vi "v0.01.vi"() -> ()   [LabVIEW 2021]
uses:
  C/Program Files/National Instruments/LabVIEW 2024/instr.lib/lvserial/lvserial.lvlib
panel:
  out "XY Graph":cluster{"X":dbl, "Y":dbl}[](graph)
  out "Imag":i32[](array[numeric])
  out "Real":i32[](array[numeric])
  out "F":dbl[](array[numeric])
  out "x/y":dbl
  in  "Step":i32
  in  "Stop":i32
  in  "Start":i32
  out "Array 3":string[](array[string])
  out "string read":string
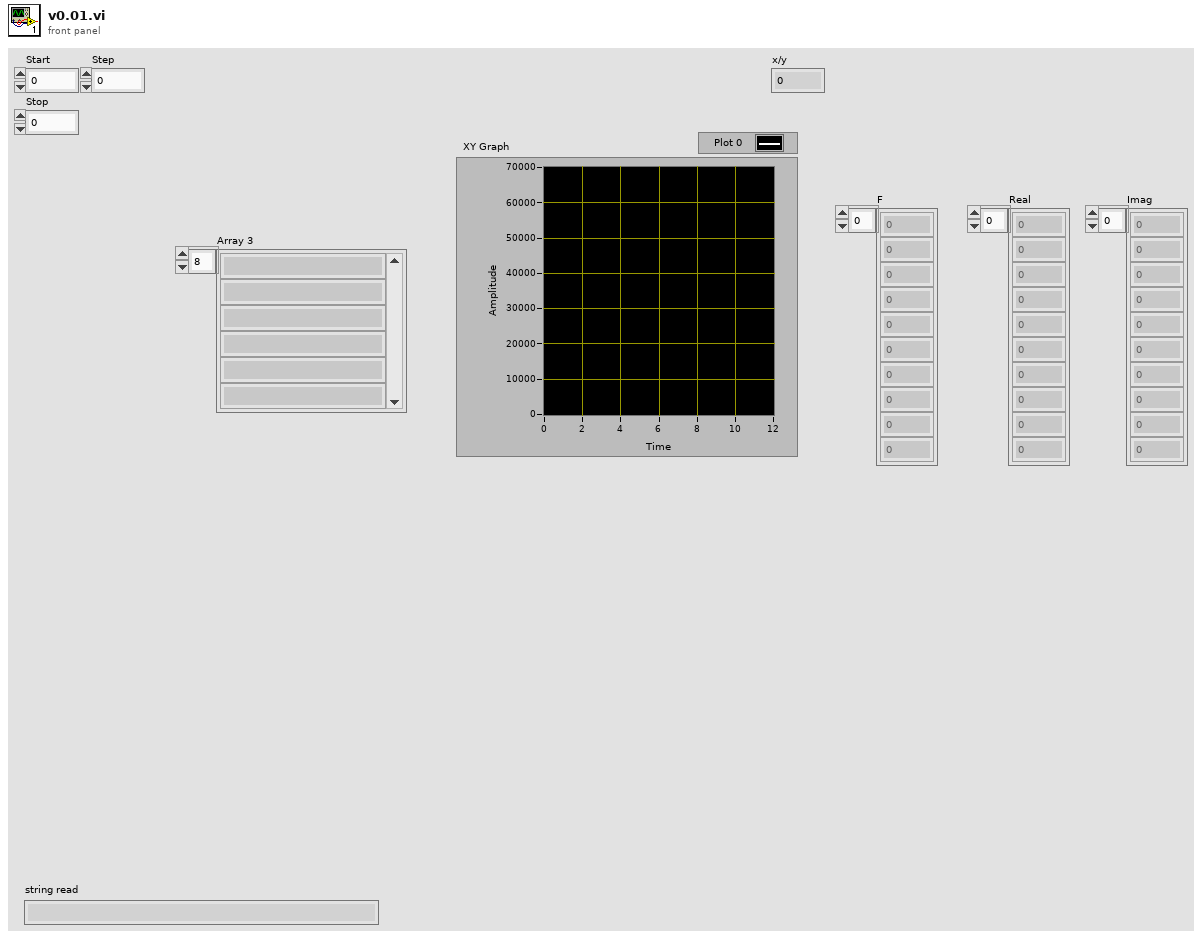
[diagram p1: front panel]
types:
  T1 = cluster{"Baud Rate":u32, "Data Bits":u16, "Parity":u16, "Stop Bits":u16}
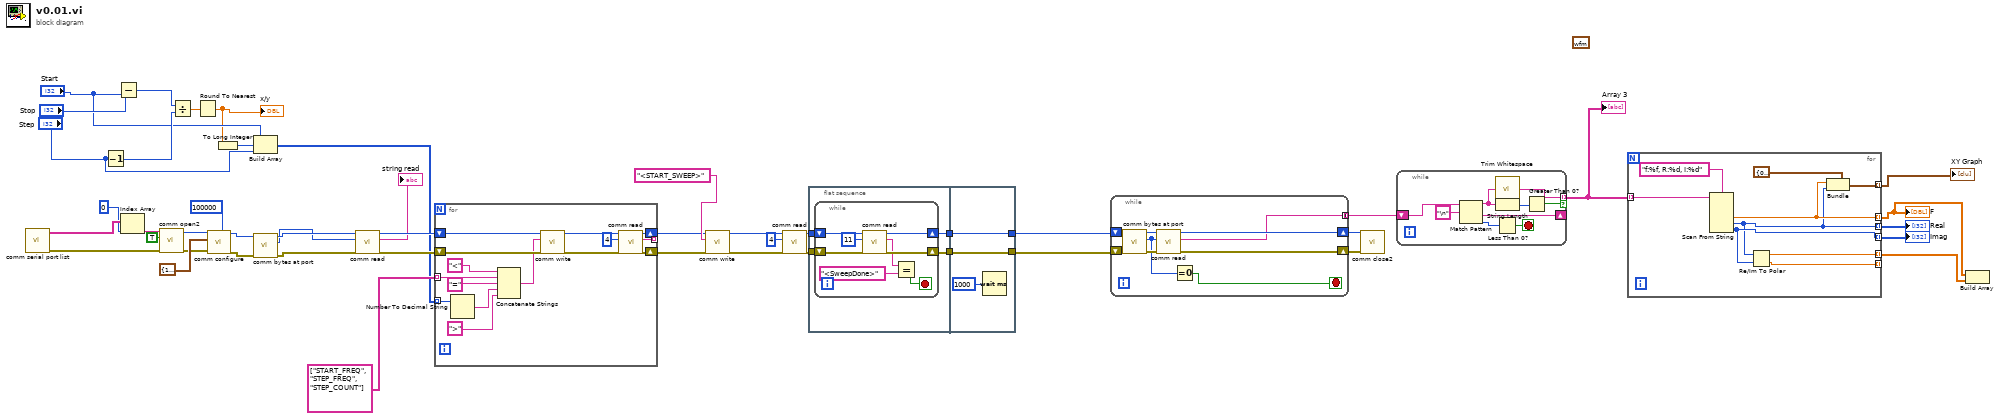
[diagram p0: block diagram]
diagram:
  (unwired) waveform(dbl) {"t0"=timestamp(0 s since 1904-01-01), "dt"=1.0, "Y"=[]} ("Waveform")
  n1 = call "comm serial port list.vi"() -> ("error out"=w45:errorcluster, "serial ports"=w43:string[])  [unwired: 10 in]
  n2 = Decrement(x="Step") -> (x-1=w14:i32)
  n3 = Subtract(x="Stop", y="Start") -> (x-y=w15:i32)
  n4 = Index Array(array=w43, index=0) -> (element=w42:string)
  n5 = call "comm open2.vi"("error in (no error)"=w45, "open duplicate?"=TRUE, "Comm Port Name"=w42) -> ("error out"=w44:errorcluster, "Comm Handle"=w46:u64)  [unwired: 2 in, 1 out]
  n6 = Divide(x=w15, y=w14) -> (x/y=w13:dbl)
  n7 = Round To Nearest(number=w13) -> (nearest integer value=w11:dbl)
  "x/y" <- w11
  n8 = call "comm configure.vi"("timeout (10000ms)"=u32 100000, "error in (no error)"=w44, "serial settings"=T1 {"Baud Rate"=115200, "Data Bits"=8, "Parity"=0, "Stop Bits"=10}, "Comm Handle"=w46) -> ("error out"=w32:errorcluster, "dup Comm Handle"=w33:u64)  [unwired: 6 in]
  n9 = To Long Integer(number=w11) -> (32bit integer=w9:i32)
  n10 = call "comm bytes at port.vi"("error in (no error)"=w32, "Comm Handle"=w33) -> ("error out"=w30:errorcluster, "bytes at port"=w29:u32, "dup Comm Handle"=w31:u64)  [unwired: 7 in]
  n11 = Build Array("Start", w9, "Step") -> (w8:i32[])
  n12 = call "comm read.vi"("error in (no error)"=w30, "requested byte count"=w29, "Comm Handle"=w31) -> ("error out"=w36:errorcluster, "string read"=→"string read":string, "dup Comm Handle"=w37:u64)  [unwired: 5 in, 1 out]
  n13 = for {
    tunnel: [w58] -> _ mode=indexing
    shift-right: [w60] -> w25
    shift-left: w37 -> [w57]
    shift-right: [w59] -> w48
    shift-left: w36 -> [w56]
    tunnel: string[] ["START_FREQ", "STEP_FREQ", "STEP_COUNT"] -> [w55] mode=indexing
    tunnel: w8 -> [w53] mode=indexing
    n14 = Number To Decimal String(number=w53) -> (decimal integer string=w50:string)  [unwired: 1 in]
    n15 = Concatenate Strings("<", w55, "=", w50, ">") -> (w52:string)
    n16 = call "comm write.vi"("error in (no error)"=w56, "string to write"=w52, "Comm Handle"=w57) -> ("error out"=w61:errorcluster, "dup Comm Handle"=w63:u64)  [unwired: 6 in, 1 out]
    n17 = call "comm read.vi"("error in (no error)"=w61, "requested byte count"=u32 4, "Comm Handle"=w63) -> ("error out"=w59:errorcluster, "string read"=w58:string, "dup Comm Handle"=w60:u64)  [unwired: 5 in, 1 out]
  }
  n18 = call "comm write.vi"("error in (no error)"=w48, "string to write"="<START_SWEEP>", "Comm Handle"=w25) -> ("error out"=w28:errorcluster, "dup Comm Handle"=w23:u64)  [unwired: 6 in, 1 out]
  n19 = call "comm read.vi"("error in (no error)"=w28, "requested byte count"=u32 4, "Comm Handle"=w23) -> ("error out"=w24:errorcluster, "dup Comm Handle"=w20:u64)  [unwired: 5 in, 2 out]
  n20 = flat-sequence {
    tunnel: w24 -> [w67]
    tunnel: w20 -> [w65]
    tunnel: [w66] -> w18
    tunnel: [w64] -> w17
    tunnel: [w77] -> w19
    tunnel: [w78] -> w21
    tunnel: w18 -> [w78]
    tunnel: w17 -> [w77]
    frame #0 {
      n21 = while {
        shift-right: [w74] -> w66
        shift-left: w67 -> [w75]
        shift-right: [w72] -> w64
        shift-left: w65 -> [w73]
        stop <- w71 stop-if-true
        n22 = call "comm read.vi"("error in (no error)"=w75, "requested byte count"=u32 11, "Comm Handle"=w73) -> ("error out"=w74:errorcluster, "string read"=w70:string, "dup Comm Handle"=w72:u64)  [unwired: 5 in, 1 out]
        n23 = Equal?(x=w70, y="<SweepDone>") -> (x = y?=w71:bool)
      }
    }
    frame #1 {
      n24 = Wait (ms)(milliseconds to wait=u32 1000) -> ()  [unwired: 1 out]
    }
  }
  n25 = while {
    shift-right: [w83] -> w27
    shift-left: w19 -> [w85]
    shift-right: [w82] -> w26
    shift-left: w21 -> [w84]
    tunnel: [w79] -> w4 mode=concatenating
    stop <- w81 stop-if-true
    n26 = call "comm bytes at port.vi"("error in (no error)"=w84, "Comm Handle"=w85) -> ("error out"=w86:errorcluster, "bytes at port"=w80:u32, "dup Comm Handle"=w87:u64)  [unwired: 7 in]
    n27 = call "comm read.vi"("error in (no error)"=w86, "requested byte count"=w80, "Comm Handle"=w87) -> ("error out"=w82:errorcluster, "string read"=w79:string, "dup Comm Handle"=w83:u64)  [unwired: 5 in, 1 out]
    n28 = Equal To 0?(x=w80) -> (x = 0?=w81:bool)
  }
  n29 = call "comm close2.vi"("error in (no error)"=w26, "Comm Handle"=w27) -> ()  [unwired: 5 in, 1 out]
  n30 = while {
    shift-right: [w92] -> _
    shift-left: w4 -> [w96]
    tunnel: [w88] -> w7 mode=indexing if=w89
    stop <- w94 stop-if-true
    n31 = Match Pattern(string=w96, regular expression="\n") -> (before substring=w91:string, after substring=w92:string, offset past match=w93:i32)  [unwired: 1 in, 1 out]
    n32 = call <vilib>:"Trim Whitespace.vi"("string"=w91) -> ("trimmed string"=w88:string)  [unwired: 1 in]
    n33 = String Length(string=w91) -> (length=w90:i32)
    n34 = Less Than 0?(x=w93) -> (x < 0?=w94:bool)
    n35 = Greater Than 0?(x=w90) -> (x > 0?=w89:bool)
  }
  "Array 3" <- w7
  n36 = for {
    tunnel: w7 -> [w104] mode=indexing
    tunnel: [w99] -> w3 mode=indexing
    tunnel: [w98] -> w6 mode=indexing
    tunnel: [w103] -> w5 mode=indexing
    tunnel: [w102] -> w2 mode=indexing
    tunnel: [w101] -> _ mode=indexing
    tunnel: [w97] -> w1 mode=indexing
    n37 = Scan From String(format string="f:%f, R:%d, I:%d", input string=w104) -> (output 1=w99:dbl, output 2=w98:i32, output 3=w103:i32)  [unwired: 5 in, 3 out]
    n38 = Re/Im To Polar(2:w103, 3:w98) -> (0:w101:dbl, 1:w102:dbl)
    n39 = Bundle(cluster=cluster{"X":dbl, "Y":dbl} {"X"=0.0, "Y"=0.0}, "X"=w99, "Y"=w98) -> (w97:cluster{"X":dbl, "Y":dbl})
  }
  "F" <- w3
  "Real" <- w6
  "Imag" <- w5
  "XY Graph" <- w1
  n40 = Build Array(w3, w2) -> ()  [unwired: 1 out]
